vi "IsMouseWithinCTRL.vi"(6 "鼠标坐标":T1={"Horizontal"=200, "Vertical"=200}, 8 "x-y":T1={"Horizontal"=100, "Vertical"=100} caption="鼠标-图例", 9 "图例边界":T2={"Width"=100, "Height"=100}, 10 "控件边界":T2={"Width"=500, "Height"=400}, 11 "控件位置":T3) -> (3 "IsMouseWithin":bool)   [LabVIEW 2012, in "WaveGraphX.xctl"]
doc: "在图例移动过程中,判断是否将图例移动出了波形图控件的范围."
uses:
  <vilib>/Utility/miscctls.llb/LVPositionTypeDef.ctl
  <vilib>/Utility/miscctls.llb/LVBoundsTypeDef.ctl
  <vilib>/Utility/miscctls.llb/LVPoint32TypeDef.ctl
  WaveGraphX.xctl
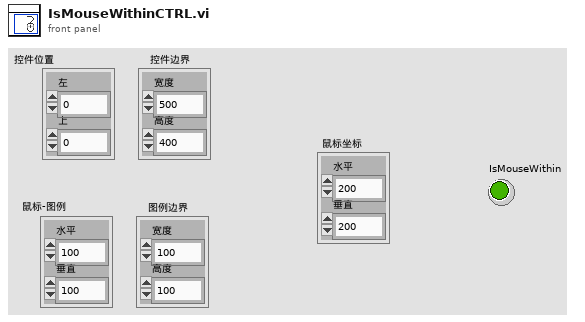
[diagram p1: front panel]
types:
  T1 = typedef "LVPoint32TypeDef.ctl" = cluster{"Horizontal":i32, "Vertical":i32}
  T2 = typedef "LVBoundsTypeDef.ctl" = cluster{"Width":u32, "Height":u32}
  T3 = typedef "LVPositionTypeDef.ctl" = cluster{"Left":i32, "Top":i32}
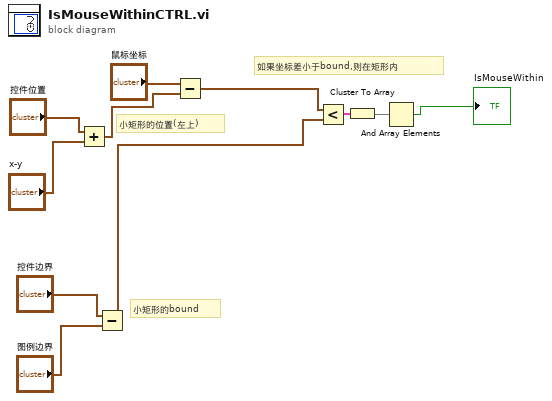
[diagram p0: block diagram]
diagram:
  # "如果坐标差小于bound,则在矩形内"
  # "小矩形的bound"
  # "小矩形的位置(左上)"
  n1 = Add(x="控件位置", y="x-y") -> (x+y=w6:T3)
  n2 = Subtract(x="控件边界", y="图例边界") -> (x-y=w4:T2)
  n3 = Subtract(x="鼠标坐标", y=w6) -> (x-y=w5:T1)
  n4 = Less?(x=w5, y=w4) -> (x < y?=w3:cluster{bool, bool})
  n5 = Cluster To Array(cluster=w3) -> (array=w2:bool[])
  n6 = And Array Elements(Boolean array=w2) -> (logical AND=→"IsMouseWithin":bool)
